vi "Polylogarithm (DBL).vi"(8 "Error In":errorcluster, 9 "n":i32, 11 "z":dbl) -> (0 "Error Out":errorcluster, 1 "Iterations":i32, 3 "Li_n(z)":dbl, 4 "Time (s)":dbl)   [LabVIEW 2021, in "Math.lvlib"]
uses:
  <vilib>/Utility/error.llb/Error Cluster From Error Code.vi
  <vilib>/ErrorRing/Error Ring.xnode
  Math.lvlib
  Time/Time.lvlib
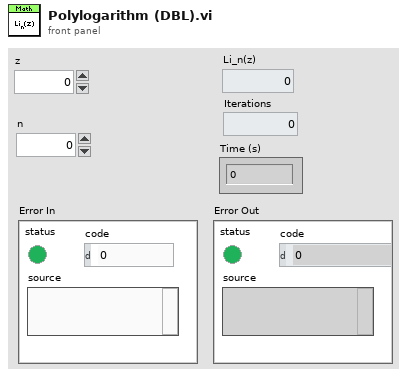
[diagram p1: front panel]
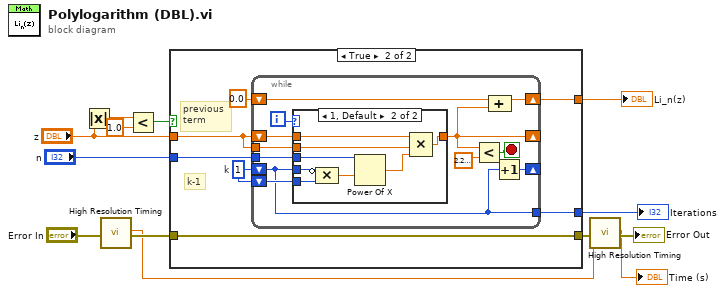
[diagram p0: block diagram]
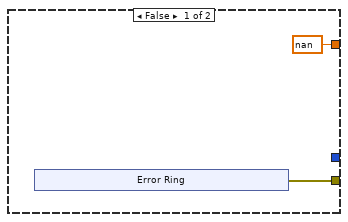
[diagram p2: hidden frame]
diagram:
  n1 = Absolute Value(x="z") -> (abs(x)=w10:dbl)
  n2 = call "High Resolution Timing.vi"("Error In"="Error In") -> ("elapsed (relative) seconds"=w2:dbl, "Error Out"=w4:errorcluster)  [unwired: 16 in, 1 out]
  n3 = Less?(x=w10, y=1.0) -> (x < y?=w8:bool)
  n4 = case shown="True" w8 {
    tunnel: "n" -> [_ w26]
    tunnel: [nan ("z") w25] -> w12
    tunnel: "z" -> [_ w23]
    tunnel: w4 -> [_ w22]
    tunnel: [w14 w22] -> w6
    tunnel: [_ w20] -> w5
    frame False {
      n5 = xnode "Error Ring"() -> ("error out"=w14:errorcluster)
    }
    frame True {
      w21 = 1  # k
      # "previous term"
      # "k-1"
      n6 = while {
        shift-right: [w30] -> _
        shift-left: w23 -> [w38]
        tunnel: w23 -> [w37]
        shift-right: [w36] -> _
        shift-left: w21 -> [w27]
        shift-left: w21 -> [w35]
        tunnel: w26 -> [w34]
        shift-right: [w29] -> w25
        shift-left: 0.0 ("z") -> [w31]
        tunnel: [w27] -> w20
        i -> [w32]
        stop <- w33 stop-if-true
        n7 = case shown="1, Default" w32 {
          tunnel: w38 -> [w39 w47]
          tunnel: w37 -> [_ w46]
          tunnel: w27 -> [_ w44]
          tunnel: w35 -> [_ w43]
          tunnel: w34 -> [_ w41]
          tunnel: [w39 w42] -> w30
          frame 0 {
          }
          frame 1, Default {
            n8 = Compound Arithmetic op=MULTIPLY(invert w44, w43) -> (w40:dbl)
            n9 = Power Of X(1:w40, 2:w41) -> (0:w45:dbl)
            n10 = Compound Arithmetic op=MULTIPLY(w47, w46, w45) -> (w42:dbl)
          }
        }
        n11 = Less?(x=w30, y=2.220446049250313e-16) -> (x < y?=w33:bool)
        n12 = Compound Arithmetic op=ADD(w31, w30) -> (w29:dbl)
        n13 = Increment(x=w27) -> (x+1=w36:i32)
      }
    }
  }
  "Li_n(z)" <- w12
  "Iterations" <- w5
  n14 = call "High Resolution Timing.vi"("relative seconds (NaN)"=w2, "Error In"=w6) -> ("elapsed (relative) seconds"=→"Time (s)":dbl, "Error Out"=→"Error Out":errorcluster)  [unwired: 15 in, 1 out]
